vi "ALTS-2015 LV2GBL Station Info.vi"(7 "Options":T4, 8 "error in":errorcluster, 10 "Station":T1, 11 "Station Cluster":T3) -> (0 "error out":errorcluster, 2 "Station Details":T1, 3 "Station Info Array":T1[](array[typedef]))   [LabVIEW 2013]
uses:
  Controls/ALTS-2015 LV2GBL Station Info Options.ctl
  Controls/ALTS-2015 Station Cluster.ctl
  Controls/ALTS-2015 Station Details.ctl
  Controls/ALTS-2015 Status Ring Indicator.ctl
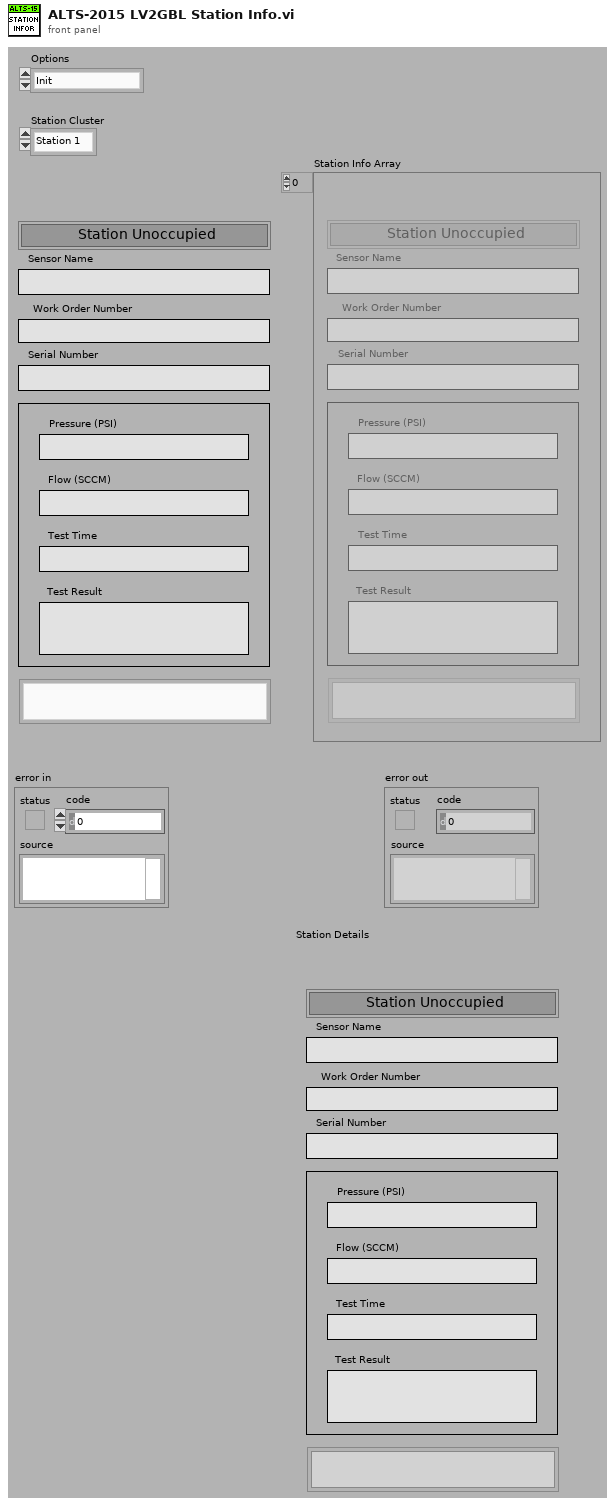
[diagram p1: front panel]
types:
  T1 = typedef "ALTS-2015 Station Details.ctl" = cluster{"Station Number":string, "Work Order Number":string, "Sensor Name":string, "Pressure (PSI)":string, "Flow (SCCM)":string, "Test Time ":string, "Test Result":string, "Serial Number":string, "Station Status":T2, "Station Occupied?":bool, "Rerun Count":i32, "Test Type":i32}
  T2 = typedef "ALTS-2015 Status Ring Indicator.ctl" = u16
  T3 = typedef "ALTS-2015 Station Cluster.ctl" = enum16{"Station 1", "Station 2", "Station 3", "Station 4"}
  T4 = typedef "ALTS-2015 LV2GBL Station Info Options.ctl" = enum16{"Init", "Read", "Read All", "Write Sensor ID", "Write  Work Order", "Write Serial Number", "Write Test Data", "Write Station Status", "Write Station Occupancy", "Write Station Test Type", "Write Rerun", "Clear All", "Clear Test Result"}
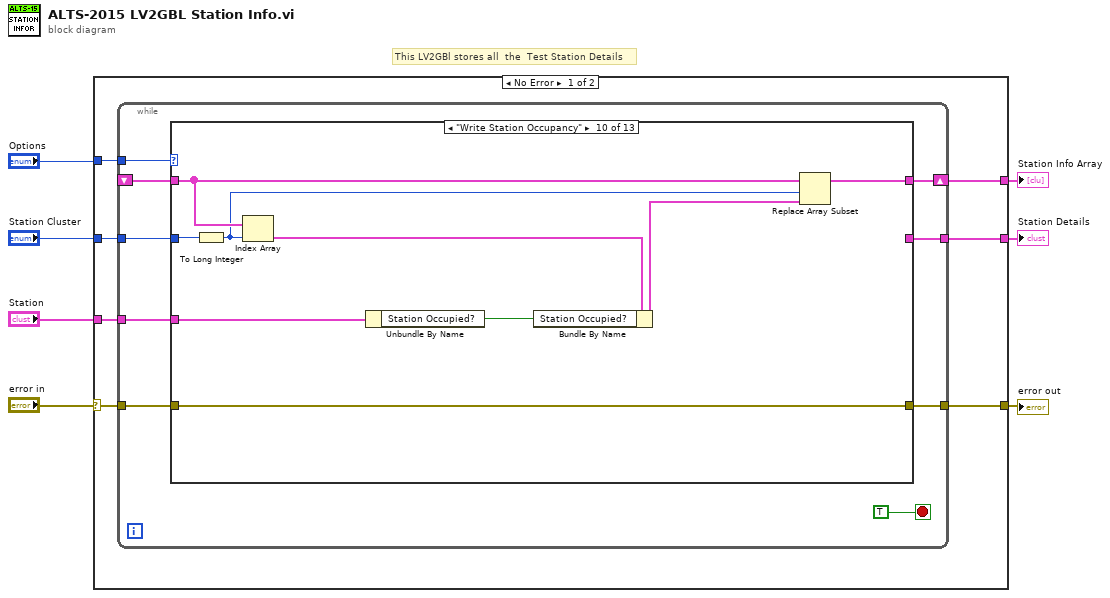
[diagram p0: block diagram]
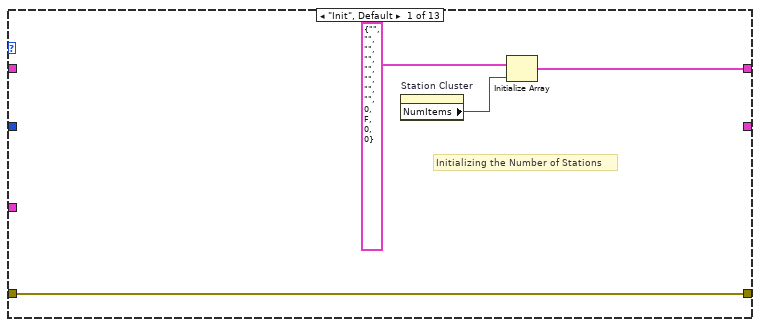
[diagram p2: hidden frame]
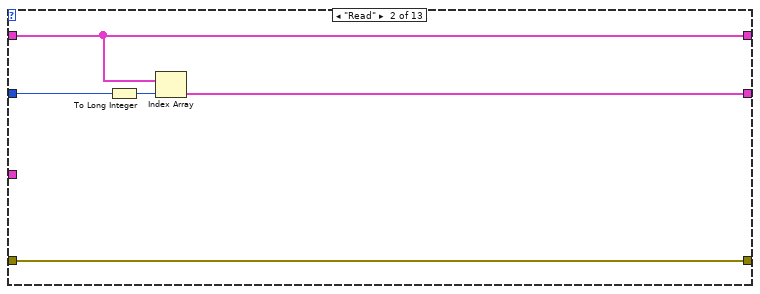
[diagram p3: hidden frame]
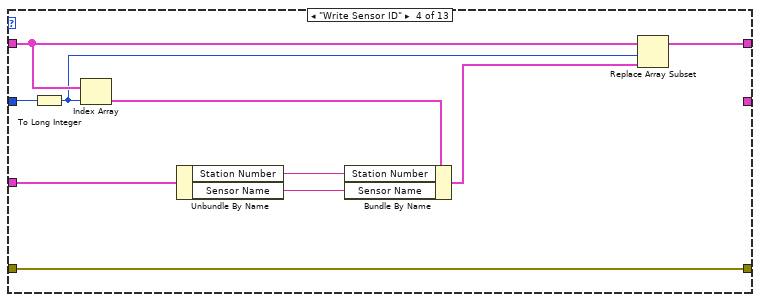
[diagram p5: hidden frame]
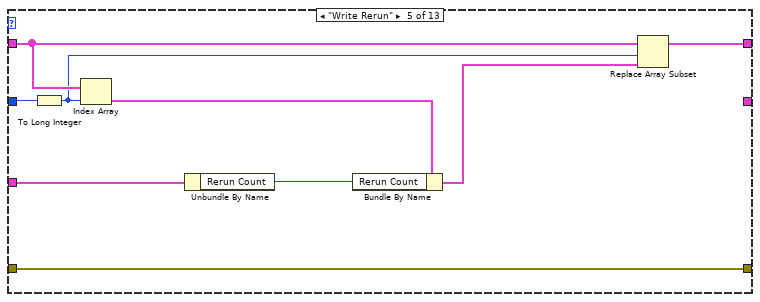
[diagram p6: hidden frame]
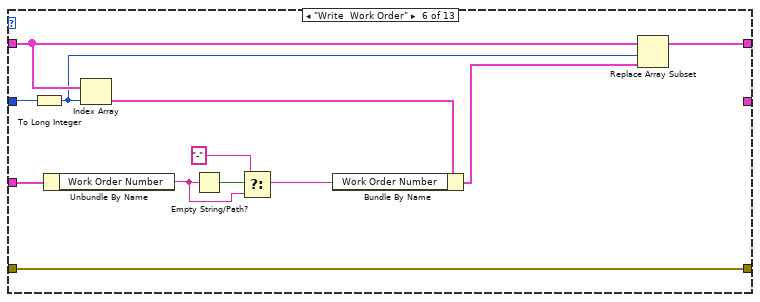
[diagram p7: hidden frame]
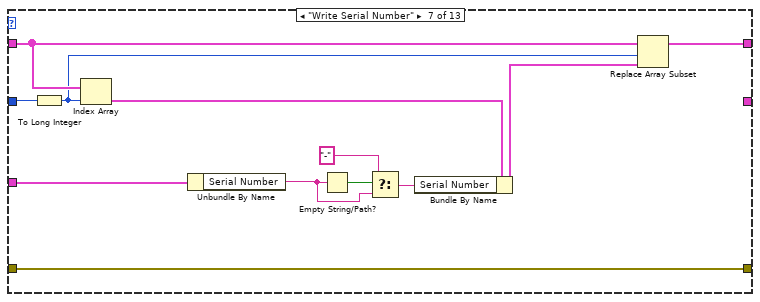
[diagram p8: hidden frame]
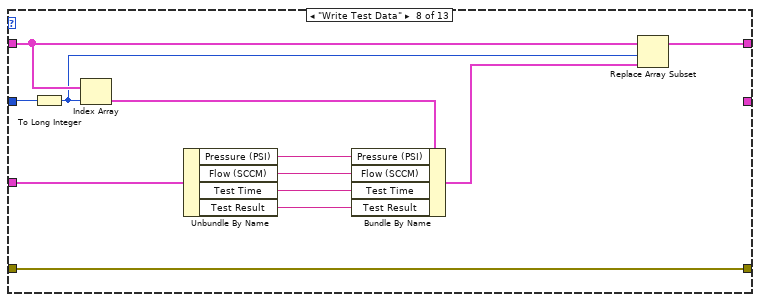
[diagram p9: hidden frame]
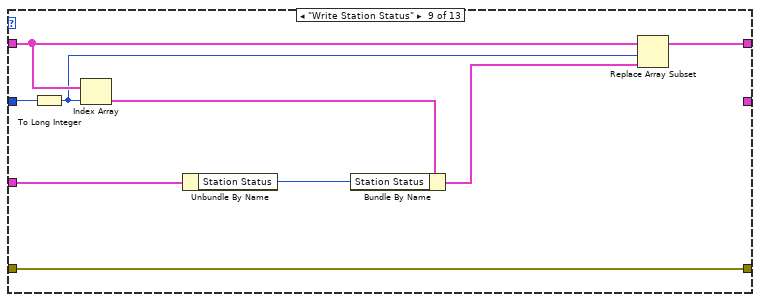
[diagram p10: hidden frame]
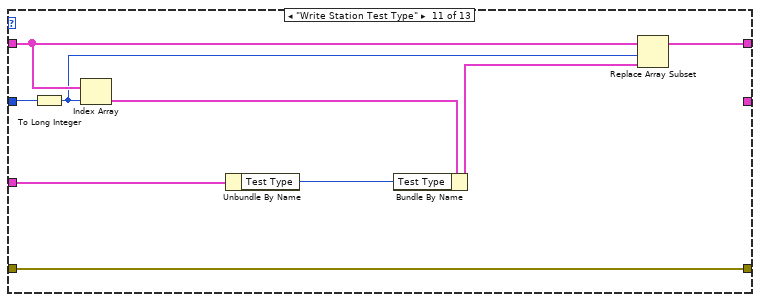
[diagram p11: hidden frame]
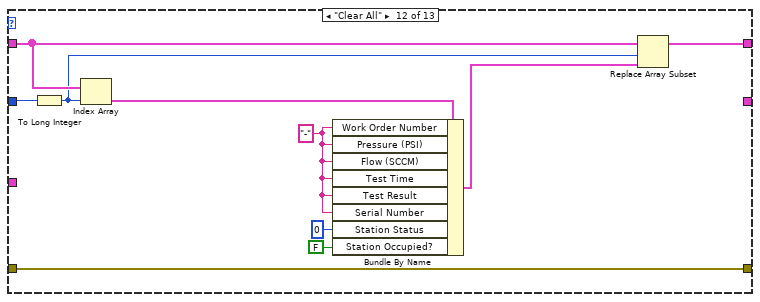
[diagram p12: hidden frame]
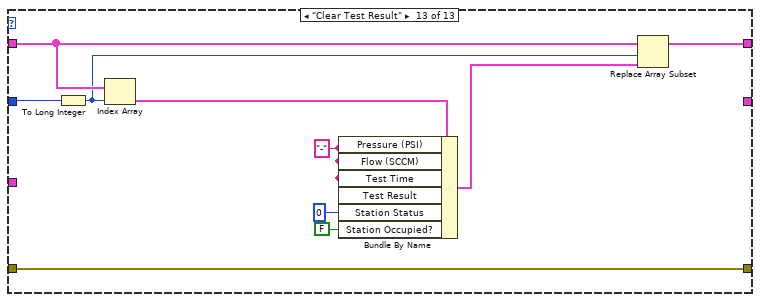
[diagram p13: hidden frame]
diagram:
  # "This LV2GBl stores all  the  Test Station Details"
  n1 = case shown="No Error" "error in" {
    selector: "error in" -> [w11 w137]
    tunnel: "Station Cluster" -> [w14 _]
    tunnel: [w13 w137] -> w7
    tunnel: "Options" -> [w12 _]
    tunnel: [w10 _] -> w3
    tunnel: "Station" -> [w9 _]
    tunnel: [w8 _] -> w1
    frame No Error {
      n2 = while {
        tunnel: w14 -> [w23]
        tunnel: [w22] -> w13
        tunnel: w12 -> [w21]
        tunnel: w11 -> [w20]
        shift-right: [w18] -> w10
        shift-left: _ -> [w17]
        tunnel: w9 -> [w16]
        tunnel: [w15] -> w8
        stop <- TRUE stop-if-true
        n3 = case shown="\"Write Station Occupancy\"" w21 {
          tunnel: w23 -> [_ w30 _ w42 w51 w63 w75 w87 w96 w105 w114 w124 w134]
          tunnel: w20 -> [w27 w32 w34 w44 w53 w65 w77 w89 w98 w107 w116 w126 w136]
          tunnel: [w27 w32 w34 w44 w53 w65 w77 w89 w98 w107 w116 w126 w136] -> w22
          tunnel: [w24 w29 w33 w38 w48 w60 w72 w83 w93 w102 w111 w122 w132] -> w18
          tunnel: w17 -> [_ w29 w33 w43 w52 w64 w76 w88 w97 w106 w115 w125 w135]
          tunnel: w16 -> [_ _ _ w41 w50 w62 w74 w86 w95 w104 w113 _ _]
          tunnel: [_ w28 _ _ _ _ _ _ _ _ _ _ _] -> w15
          frame "Init", Default {
            # "Initializing the Number of Stations"
            n4 = property on="Station Cluster" class="Enum (strict)"() -> ("NumItems"=w25:u32)  [unwired: 2 in, 2 out]
            n5 = Initialize Array(T1 {"Station Number"="", "Work Order Number"="", "Sensor Name"="", "Pressure (PSI)"="", "Flow (SCCM)"="", "Test Time "="", "Test Result"="", "Serial Number"="", "Station Status"=0, "Station Occupied?"=FALSE, "Rerun Count"=0, "Test Type"=0} ("Station 1"), w25) -> (w24:T1[])
          }
          frame "Read" {
            n6 = To Long Integer(number=w30) -> (32bit integer=w31:i32)
            n7 = Index Array(array=w29, index=w31) -> (element=w28:T1)
          }
          frame "Read All" {
          }
          frame "Write Sensor ID" {
            n8 = To Long Integer(number=w42) -> (32bit integer=w37:i32)
            n9 = Index Array(array=w43, index=w37) -> (element=w40:T1)
            n10 = Unbundle By Name(w41) -> ("Station Number"=w35:string, "Sensor Name"=w39:string)
            n11 = Bundle By Name(cluster=w40, "Station Number"=w35, "Sensor Name"=w39) -> (w36:T1)
            n12 = Replace Array Subset(array=w43, new element=w36, index=w37) -> (w38:T1[])
          }
          frame "Write Rerun" {
            n13 = To Long Integer(number=w51) -> (32bit integer=w47:i32)
            n14 = Index Array(array=w52, index=w47) -> (element=w49:T1)
            n15 = Unbundle By Name(w50) -> ("Rerun Count"=w45:i32)
            n16 = Bundle By Name(cluster=w49, "Rerun Count"=w45) -> (w46:T1)
            n17 = Replace Array Subset(array=w52, new element=w46, index=w47) -> (w48:T1[])
          }
          frame "Write  Work Order" {
            n18 = To Long Integer(number=w63) -> (32bit integer=w59:i32)
            n19 = Unbundle By Name(w62) -> ("Work Order Number"=w56:string)
            n20 = Index Array(array=w64, index=w59) -> (element=w61:T1)
            n21 = Empty String/Path?(string/path=w56) -> (empty?=w57:bool)
            n22 = Select(t="-", s=w57, f=w56) -> (s? t:f=w54:string)
            n23 = Bundle By Name(cluster=w61, "Work Order Number"=w54) -> (w58:T1)
            n24 = Replace Array Subset(array=w64, new element=w58, index=w59) -> (w60:T1[])
          }
          frame "Write Serial Number" {
            n25 = To Long Integer(number=w75) -> (32bit integer=w71:i32)
            n26 = Index Array(array=w76, index=w71) -> (element=w73:T1)
            n27 = Unbundle By Name(w74) -> ("Serial Number"=w68:string)
            n28 = Empty String/Path?(string/path=w68) -> (empty?=w69:bool)
            n29 = Select(t="-", s=w69, f=w68) -> (s? t:f=w66:string)
            n30 = Bundle By Name(cluster=w73, "Serial Number"=w66) -> (w70:T1)
            n31 = Replace Array Subset(array=w76, new element=w70, index=w71) -> (w72:T1[])
          }
          frame "Write Test Data" {
            n32 = To Long Integer(number=w87) -> (32bit integer=w82:i32)
            n33 = Index Array(array=w88, index=w82) -> (element=w85:T1)
            n34 = Unbundle By Name(w86) -> ("Pressure (PSI)"=w84:string, "Flow (SCCM)"=w78:string, "Test Time"=w79:string, "Test Result"=w80:string)
            n35 = Bundle By Name(cluster=w85, "Pressure (PSI)"=w84, "Flow (SCCM)"=w78, "Test Time"=w79, "Test Result"=w80) -> (w81:T1)
            n36 = Replace Array Subset(array=w88, new element=w81, index=w82) -> (w83:T1[])
          }
          frame "Write Station Status" {
            n37 = To Long Integer(number=w96) -> (32bit integer=w92:i32)
            n38 = Index Array(array=w97, index=w92) -> (element=w94:T1)
            n39 = Unbundle By Name(w95) -> ("Station Status"=w90:T2)
            n40 = Bundle By Name(cluster=w94, "Station Status"=w90) -> (w91:T1)
            n41 = Replace Array Subset(array=w97, new element=w91, index=w92) -> (w93:T1[])
          }
          frame "Write Station Occupancy" {
            n42 = To Long Integer(number=w105) -> (32bit integer=w101:i32)
            n43 = Index Array(array=w106, index=w101) -> (element=w103:T1)
            n44 = Unbundle By Name(w104) -> ("Station Occupied?"=w99:bool)
            n45 = Bundle By Name(cluster=w103, "Station Occupied?"=w99) -> (w100:T1)
            n46 = Replace Array Subset(array=w106, new element=w100, index=w101) -> (w102:T1[])
          }
          frame "Write Station Test Type" {
            n47 = To Long Integer(number=w114) -> (32bit integer=w110:i32)
            n48 = Index Array(array=w115, index=w110) -> (element=w112:T1)
            n49 = Unbundle By Name(w113) -> ("Test Type"=w108:i32)
            n50 = Bundle By Name(cluster=w112, "Test Type"=w108) -> (w109:T1)
            n51 = Replace Array Subset(array=w115, new element=w109, index=w110) -> (w111:T1[])
          }
          frame "Clear All" {
            w119 = "-" ("Work Order Number")
            n52 = To Long Integer(number=w124) -> (32bit integer=w121:i32)
            n53 = Index Array(array=w125, index=w121) -> (element=w123:T1)
            n54 = Bundle By Name(cluster=w123, "Work Order Number"=w119, "Pressure (PSI)"=w119, "Flow (SCCM)"=w119, "Test Time"=w119, "Test Result"=w119, "Serial Number"=w119, "Station Status"=T2 0, "Station Occupied?"=FALSE) -> (w120:T1)
            n55 = Replace Array Subset(array=w125, new element=w120, index=w121) -> (w122:T1[])
          }
          frame "Clear Test Result" {
            w129 = "-" ("Work Order Number")
            n56 = To Long Integer(number=w134) -> (32bit integer=w131:i32)
            n57 = Index Array(array=w135, index=w131) -> (element=w133:T1)
            n58 = Bundle By Name(cluster=w133, "Pressure (PSI)"=w129, "Flow (SCCM)"=w129, "Test Time"=w129, "Test Result"=w129, "Station Status"=T2 0 ("Station Occupied?"), "Station Occupied?"=FALSE) -> (w130:T1)
            n59 = Replace Array Subset(array=w135, new element=w130, index=w131) -> (w132:T1[])
          }
        }
      }
    }
    frame Error {
    }
  }
  "error out" <- w7
  "Station Info Array" <- w3
  "Station Details" <- w1
